vi "Caculate 2D Arr Rotate.vi"(10 "Laser Point 2D Arr":cluster{"X":sgl, "Y":sgl, "Z":sgl}[][](array[cluster]), 11 "Mark Data":T1) -> (2 "New Laser Point":cluster{dbl, dbl}[][](array[cluster]), 3 "Panel Rotate Angle":dbl)   [LabVIEW 2019]
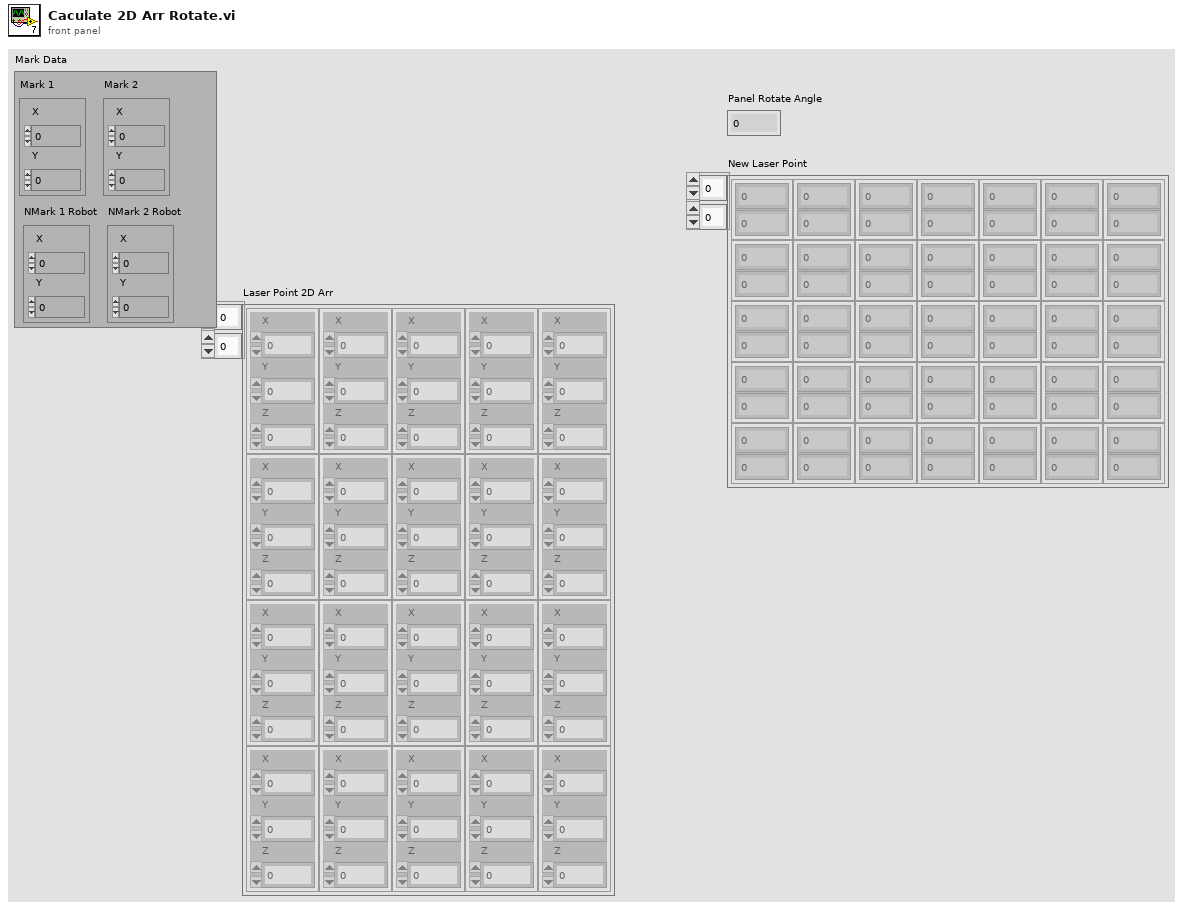
[diagram p1: front panel]
types:
  T1 = cluster{"Mark 1":cluster{"X":dbl, "Y":dbl}, "Mark 2":cluster{"X":dbl, "Y":dbl}, "NMark 1 Robot":cluster{"X":dbl, "Y":dbl}, "NMark 2 Robot":cluster{"X":dbl, "Y":dbl}}
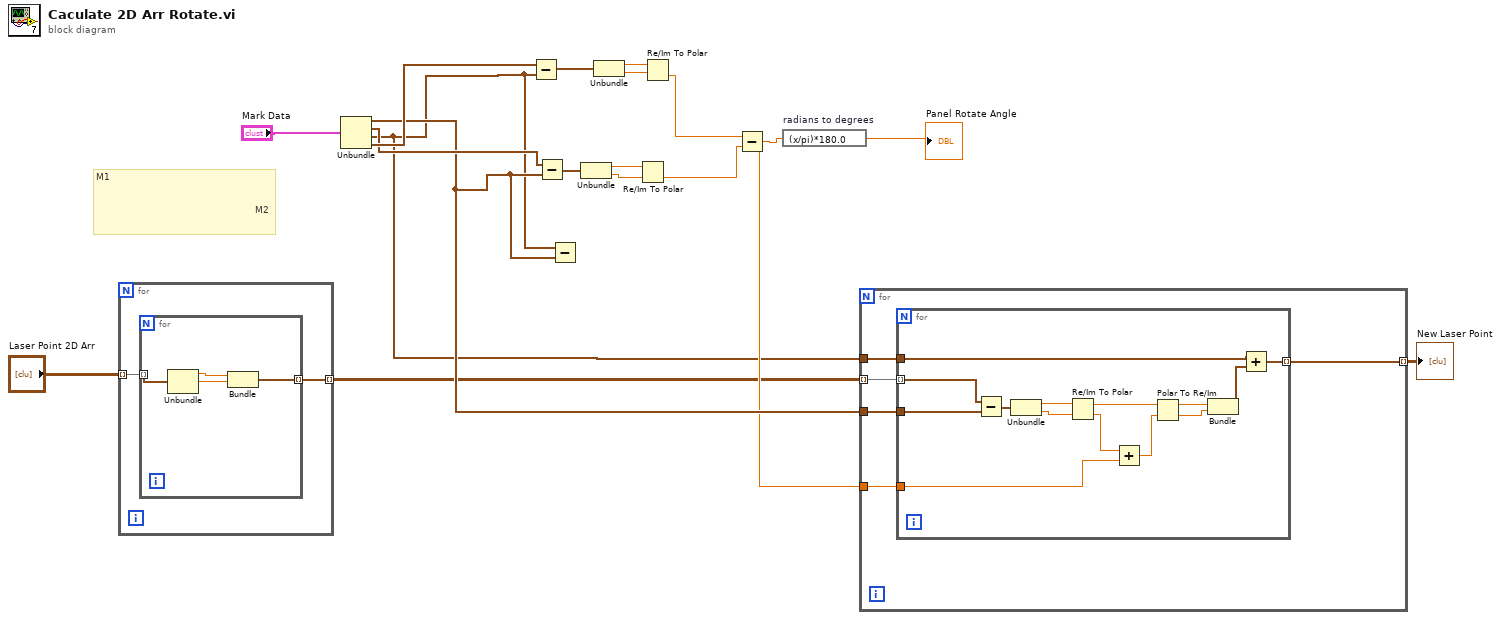
[diagram p0: block diagram]
diagram:
  # "M1                                       \n\n\n                                                     M2"
  n1 = for {
    tunnel: "Laser Point 2D Arr" -> [w20] mode=indexing
    tunnel: [w19] -> w2 mode=indexing
    n2 = for {
      tunnel: w20 -> [w24] mode=indexing
      tunnel: [w21] -> w19 mode=indexing
      n3 = Unbundle(w24) -> ("X"=w23:sgl, "Y"=w22:sgl)  [unwired: 1 out]
      n4 = Bundle("X"=w23, "Y"=w22) -> (w21:cluster{"X":sgl, "Y":sgl})  [unwired: 1 in]
    }
  }
  n5 = Unbundle("Mark Data") -> ("Mark 1"=w6:cluster{"X":dbl, "Y":dbl}, "Mark 2"=w7:cluster{"X":dbl, "Y":dbl}, "NMark 1 Robot"=w1:cluster{"X":dbl, "Y":dbl}, "NMark 2 Robot"=w8:cluster{"X":dbl, "Y":dbl})
  n6 = Subtract(x=w8, y=w1) -> (x-y=w12:cluster{"X":dbl, "Y":dbl})
  n7 = Subtract(x=w7, y=w6) -> (x-y=w11:cluster{"X":dbl, "Y":dbl})
  n8 = Subtract(x=w1, y=w6) -> ()  [unwired: 1 out]
  n9 = Unbundle(w11) -> ("X"=w15:dbl, "Y"=w16:dbl)
  n10 = Unbundle(w12) -> ("X"=w13:dbl, "Y"=w14:dbl)
  n11 = Re/Im To Polar(2:w16, 3:w15) -> (0:w18:dbl)  [unwired: 1 out]
  n12 = Re/Im To Polar(2:w14, 3:w13) -> (0:w17:dbl)  [unwired: 1 out]
  n13 = Subtract(x=w17, y=w18) -> (x-y=w5:dbl)
  n14 = expression code="(x/pi)*180.0" "radians to degrees"(w5) -> (→"Panel Rotate Angle":dbl)
  n15 = for {
    tunnel: w2 -> [w29] mode=indexing
    tunnel: w6 -> [w28]
    tunnel: w5 -> [w27]
    tunnel: w1 -> [w26]
    tunnel: [w25] -> w10 mode=indexing
    n16 = for {
      tunnel: w29 -> [w43] mode=indexing
      tunnel: w28 -> [w42]
      tunnel: w27 -> [w37]
      tunnel: w26 -> [w32]
      tunnel: [w30] -> w25 mode=indexing
      n17 = Subtract(x=w43, y=w42) -> (x-y=w39:cluster{"X":dbl, "Y":dbl})
      n18 = Unbundle(w39) -> ("X"=w41:dbl, "Y"=w40:dbl)
      n19 = Re/Im To Polar(2:w40, 3:w41) -> (0:w38:dbl, 1:w36:dbl)
      n20 = Add(x=w38, y=w37) -> (x+y=w35:dbl)
      n21 = Polar To Re/Im(2:w35, 3:w36) -> (0:w33:dbl, 1:w34:dbl)
      n22 = Bundle(w34, w33) -> (w31:cluster{dbl, dbl})  [unwired: 1 in]
      n23 = Add(x=w32, y=w31) -> (x+y=w30:cluster{dbl, dbl})
    }
  }
  "New Laser Point" <- w10
